vi "DevTests_Stress.vi"() -> ()   [LabVIEW 2024]
uses:
  SDL3/Init/InitFlags--ring.ctl
  SDL3/Error/GetError-UiThread.vi
  <vilib>/Utility/error.llb/Error Cluster From Error Code.vi
  SDL3/Init/Init.lvlib
panel:
  in  "stop":bool
  out "i":i32
  out "error out":errorcluster
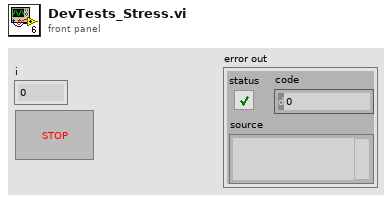
[diagram p1: front panel]
types:
  T1 = typedef "SDL3.lvlib/Init.lvlib/InitFlags--ring.ctl" = u32
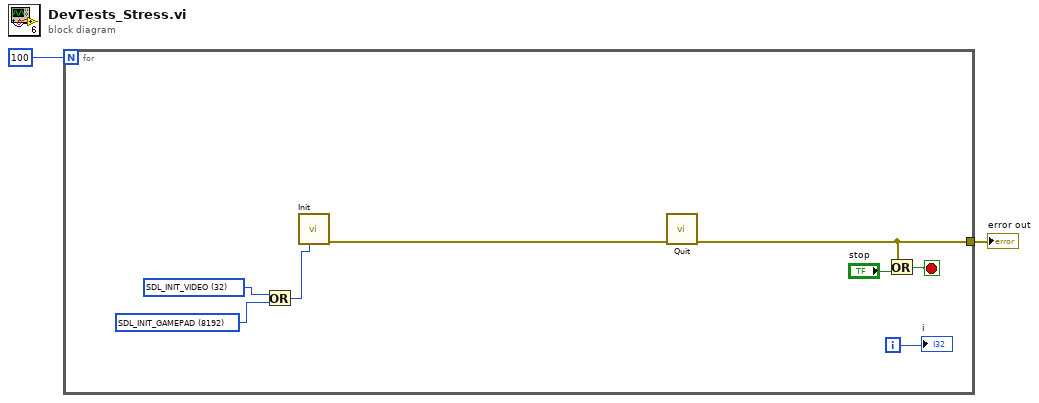
[diagram p0: block diagram]
diagram:
  n1 = for {
    N: 100 -> [_]
    tunnel: [w9] -> w1
    i -> [w3]
    stop <- w5 stop-if-true
    w7 = T1 8192 items=["NONE"=0, "SDL_INIT_AUDIO"=16, "SDL_INIT_VIDEO"=32, "SDL_INIT_JOYSTICK"=512, "SDL_INIT_HAPTIC"=4096, "SDL_INIT_GAMEPAD"=8192, "SDL_INIT_EVENTS"=16384, "SDL_INIT_SENSOR"=32768, "SDL_INIT_CAMER"=65536] ("InitFlags")
    w8 = T1 32 items=["NONE"=0, "SDL_INIT_AUDIO"=16, "SDL_INIT_VIDEO"=32, "SDL_INIT_JOYSTICK"=512, "SDL_INIT_HAPTIC"=4096, "SDL_INIT_GAMEPAD"=8192, "SDL_INIT_EVENTS"=16384, "SDL_INIT_SENSOR"=32768, "SDL_INIT_CAMER"=65536] ("InitFlags")
    n2 = Or(x=w8, y=w7) -> (x .or. y?=w6:T1)
    n3 = call "Init.vi"("InitFlags"=w6) -> ("error out"=w10:errorcluster)  [unwired: 10 in]
    n4 = call "Quit.vi"("No Error"=w10) -> ("error out"=w9:errorcluster)  [unwired: 10 in]
    n5 = Or(x=w9, y="stop") -> (x .or. y?=w5:bool)
    "i" <- w3
  }
  "error out" <- w1
